vi "Control - Generic - Lambda PID Host.vi"() -> ()   [LabVIEW 2015, in "ECS-Host.lvlib"]
uses:
  ECS-Host.lvlib
panel:
  out "IntegralEffort":sgl caption="[mg/cyc]"
  out "UEGO1Lambda":sgl caption="[]"
  in  "FuelTrim_Man":sgl caption="[]"
  in  "FuelTrim_ManE":bool
  out "FuelTrim_Des":sgl caption="[mg/cyc]"
  out "ClosedLoopFuelTrimActive":bool
  in  "ClosedLoopFuelTrim_E":bool
  in  "FuelTrim_Td":sgl caption="[]"
  in  "FuelTrim_Ti":sgl caption="[]"
  in  "FuelTrim_Kp":sgl caption="[]"
  out "FuelTrim_PIDOut":sgl caption="[mg/cyc]"
  in  "FuelTrim_PIDMin":sgl caption="[]"
  in  "FuelTrim_PIDMax":sgl caption="[mg/cyc]"
  out "Lambda_Des":sgl caption="[]"
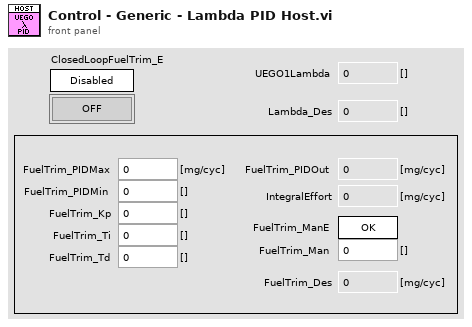
[diagram p1: front panel]
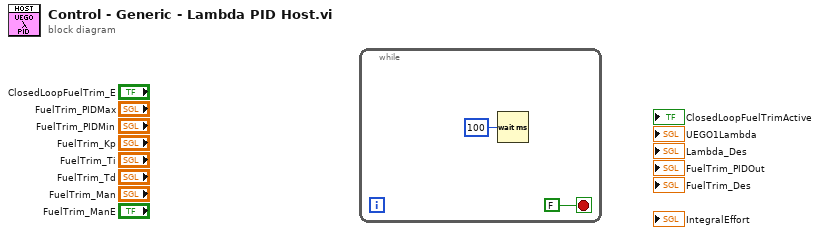
[diagram p0: block diagram]
diagram:
  n1 = while {
    stop <- FALSE stop-if-true
    n2 = Wait (ms)(milliseconds to wait=u32 100) -> ()  [unwired: 1 out]
  }
